vi "load_waypoint_icons.vi"() -> (3 "Waypoint Icon Reference":T1)   [LabVIEW 2013]
doc: "Loads the boat icon for use on the map. Also, replaces all the black pixels with transparent pixels.\n\n4/5/2014\nMac-I Crowell"
uses:
  TypeDef/waypoint_icon_references.ctl
  <vilib>/vision/Image Controls.llb/IMAQ Image.ctl
panel:
  out "Mission Image":T2(plugin-control)
  out "appended boat icon path":path
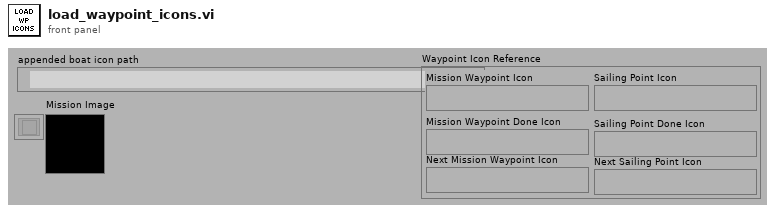
[diagram p1: front panel]
types:
  T1 = typedef "waypoint_icon_references.ctl" = cluster{"Mission Waypoint Icon":T2, "Sailing Point Icon":T2, "Mission Waypoint Done Icon":T2, "Sailing Point Done Icon":T2, "Next Mission Waypoint Icon":T2, "Next Sailing Point Icon":T2}
  T2 = typedef "IMAQ Image.ctl" = refnum<image>
  T3 = typedef "Image Type" = u32
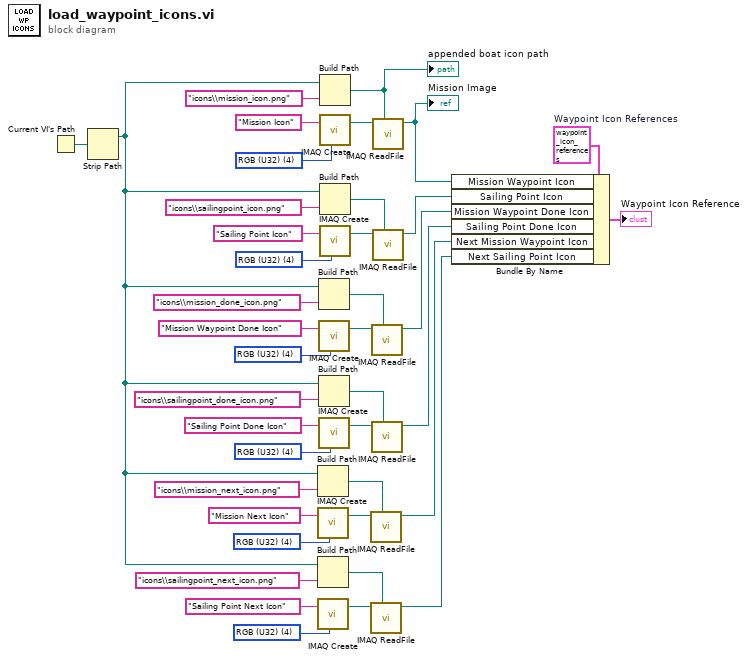
[diagram p0: block diagram]
diagram:
  w4 = T3 4 items=["Grayscale (U8)", "Grayscale (I16)", "Grayscale (SGL)", "Complex (CSG)", "RGB (U32)", "HSL (U32)", "RGB (U64)", "Grayscale (U16)"] ("Image Type")
  w13 = T3 4 items=["Grayscale (U8)", "Grayscale (I16)", "Grayscale (SGL)", "Complex (CSG)", "RGB (U32)", "HSL (U32)", "RGB (U64)", "Grayscale (U16)"] ("Image Type")
  w16 = T3 4 items=["Grayscale (U8)", "Grayscale (I16)", "Grayscale (SGL)", "Complex (CSG)", "RGB (U32)", "HSL (U32)", "RGB (U64)", "Grayscale (U16)"] ("Image Type")
  w25 = T3 4 items=["Grayscale (U8)", "Grayscale (I16)", "Grayscale (SGL)", "Complex (CSG)", "RGB (U32)", "HSL (U32)", "RGB (U64)", "Grayscale (U16)"] ("Image Type")
  w27 = T1 {"Mission Waypoint Icon"=refnum, "Sailing Point Icon"=refnum, "Mission Waypoint Done Icon"=refnum, "Sailing Point Done Icon"=refnum, "Next Mission Waypoint Icon"=refnum, "Next Sailing Point Icon"=refnum}  # Waypoint Icon References
  w30 = T3 4 items=["Grayscale (U8)", "Grayscale (I16)", "Grayscale (SGL)", "Complex (CSG)", "RGB (U32)", "HSL (U32)", "RGB (U64)", "Grayscale (U16)"] ("Image Type")
  w40 = T3 4 items=["Grayscale (U8)", "Grayscale (I16)", "Grayscale (SGL)", "Complex (CSG)", "RGB (U32)", "HSL (U32)", "RGB (U64)", "Grayscale (U16)"] ("Image Type")
  n1 = Current VI's Path() -> (path=w37:path)
  n2 = Strip Path(path=w37) -> (stripped path=w1:path)  [unwired: 1 out]
  n3 = Build Path(base path=w1, name or relative path="icons\\mission_next_icon.png") -> (appended path=w9:path)
  n4 = call "IMAQ Create"("Image Name"="Mission Next Icon", "Image Type"=w13) -> ("New Image"=w11:T2)  [unwired: 2 in, 2 out]
  n5 = Build Path(base path=w1, name or relative path="icons\\sailingpoint_next_icon.png") -> (appended path=w8:path)
  n6 = call "IMAQ Create"("Image Name"="Sailing Point Next Icon", "Image Type"=w4) -> ("New Image"=w6:T2)  [unwired: 2 in, 2 out]
  n7 = Build Path(base path=w1, name or relative path="icons\\mission_done_icon.png") -> (appended path=w21:path)
  n8 = call "IMAQ Create"("Image Name"="Mission Waypoint Done Icon", "Image Type"=w25) -> ("New Image"=w23:T2)  [unwired: 2 in, 2 out]
  n9 = Build Path(base path=w1, name or relative path="icons\\sailingpoint_done_icon.png") -> (appended path=w20:path)
  n10 = call "IMAQ Create"("Image Name"="Sailing Point Done Icon", "Image Type"=w16) -> ("New Image"=w18:T2)  [unwired: 2 in, 2 out]
  n11 = Build Path(base path=w1, name or relative path="icons\\mission_icon.png") -> (appended path=w35:path)
  "appended boat icon path" <- w35
  n12 = call "IMAQ Create"("Image Name"="Mission Icon", "Image Type"=w40) -> ("New Image"=w38:T2)  [unwired: 2 in, 2 out]
  n13 = Build Path(base path=w1, name or relative path="icons\\sailingpoint_icon.png") -> (appended path=w34:path)
  n14 = call "IMAQ Create"("Image Name"="Sailing Point Icon", "Image Type"=w30) -> ("New Image"=w32:T2)  [unwired: 2 in, 2 out]
  n15 = call "IMAQ ReadFile"("File Path"=w9, "Image"=w11) -> ("Image Out"=w3:T2)  [unwired: 3 in, 6 out]
  n16 = call "IMAQ ReadFile"("File Path"=w8, "Image"=w6) -> ("Image Out"=w2:T2)  [unwired: 3 in, 6 out]
  n17 = call "IMAQ ReadFile"("File Path"=w21, "Image"=w23) -> ("Image Out"=w14:T2)  [unwired: 3 in, 6 out]
  n18 = call "IMAQ ReadFile"("File Path"=w20, "Image"=w18) -> ("Image Out"=w15:T2)  [unwired: 3 in, 6 out]
  n19 = call "IMAQ ReadFile"("File Path"=w35, "Image"=w38) -> ("Image Out"=w29:T2)  [unwired: 3 in, 6 out]
  "Mission Image" <- w29
  n20 = call "IMAQ ReadFile"("File Path"=w34, "Image"=w32) -> ("Image Out"=w28:T2)  [unwired: 3 in, 6 out]
  n21 = Bundle By Name(cluster=w27, "Mission Waypoint Icon"=w29, "Sailing Point Icon"=w28, "Mission Waypoint Done Icon"=w14, "Sailing Point Done Icon"=w15, "Next Mission Waypoint Icon"=w3, "Next Sailing Point Icon"=w2) -> (→"Waypoint Icon Reference":T1)
